vi "COMTester_86.vi"() -> ()   [LabVIEW 2020]
panel:
  out "return count":u32
  out "VISA resource name out":refnum<visa-resource-name>
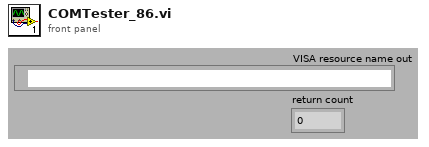
[diagram p1: front panel]
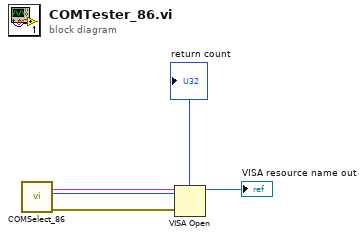
[diagram p0: block diagram]
diagram:
  n1 = call "COMSelect_86.vi"() -> ("error out"=w3:errorcluster, "return count"=→"return count":u32, "COM Port Selected"=w4:string)  [unwired: 1 in, 7 out]
  n2 = VISA Open(error in (no error)=w3, VISA resource name=w4) -> (VISA resource name=→"VISA resource name out":refnum<visa-resource-name>)  [unwired: 4 out]
